vi "ConfigAndGrabEdited.vi"() -> ()   [LabVIEW 2025]
uses:
  <vilib>/userDefined/High Color/IMAQdx.ctl
  <vilib>/vision/driver/IMAQdx.llb/IMAQdx Buffer Number Mode.ctl
  <vilib>/vision/driver/NI_Vision_Acquisition_Software.lvlib
  <resource>/objmgr/imaqdx.rc
panel:
  in  "milliseconds to wait":u32
  in  "Packet size":i64=1 min=1 step=1
  out "DeviceModelName":string
  in  "OffsetY":i64=100
  in  "Height":i64=600 min=1 max=1088 step=1
  in  "OffsetX":i64=200
  in  "Width":i64=800 min=1 max=2048 step=1
  in  "ExposureTime (ms)":dbl=850.5 min=0.0 format="%#_9f"
  in  "Camera Name":T1
  out "Frame Rate":dbl(knob) scale=0.0..100.0 scale format="%.1f"
  out "Buffer Number":u32
  out "Image":T2(plugin-control)
  in  "stop":bool
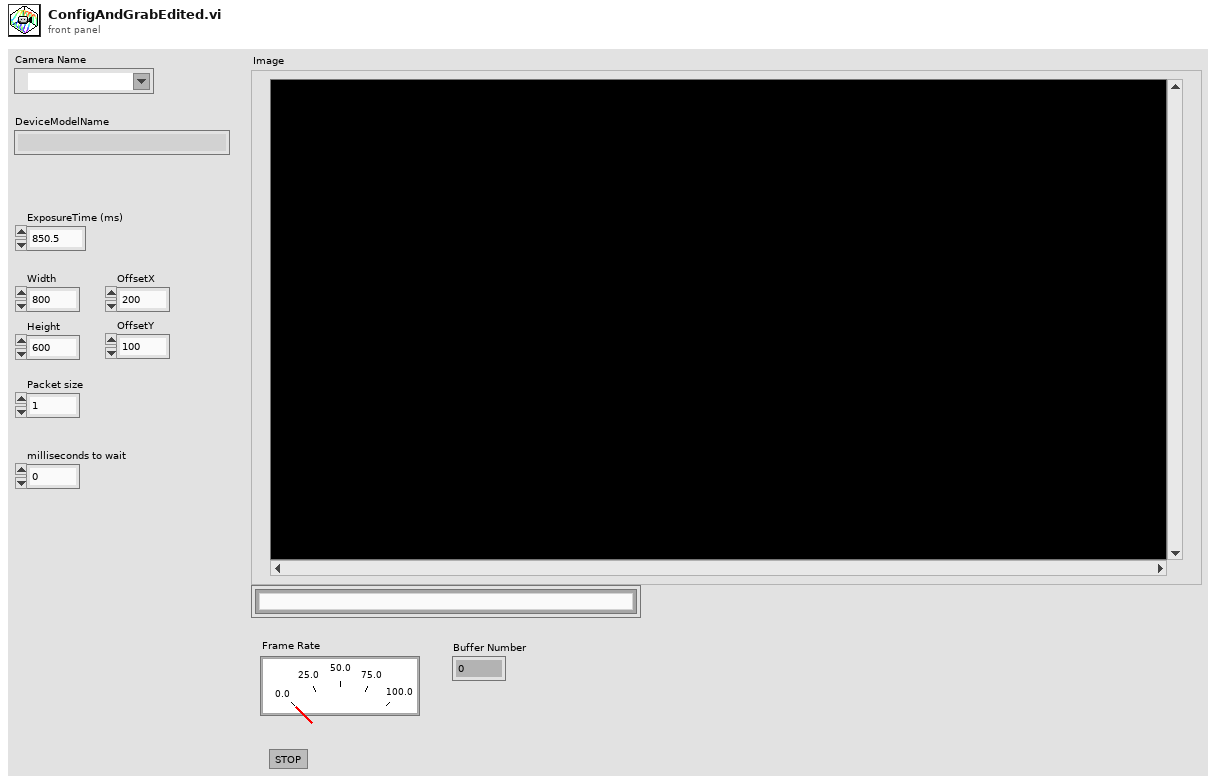
[diagram p1: front panel]
types:
  T1 = typedef "IMAQdx.ctl" = refnum<k21>
  T2 = typedef "IMAQ Image.ctl" = refnum<image>
  T3 = typedef "NI_Vision_Acquisition_Software.lvlib/IMAQdx Buffer Number Mode.ctl" = enum32{"Next", "Last", "Buffer Number", "Every", "Last New"}
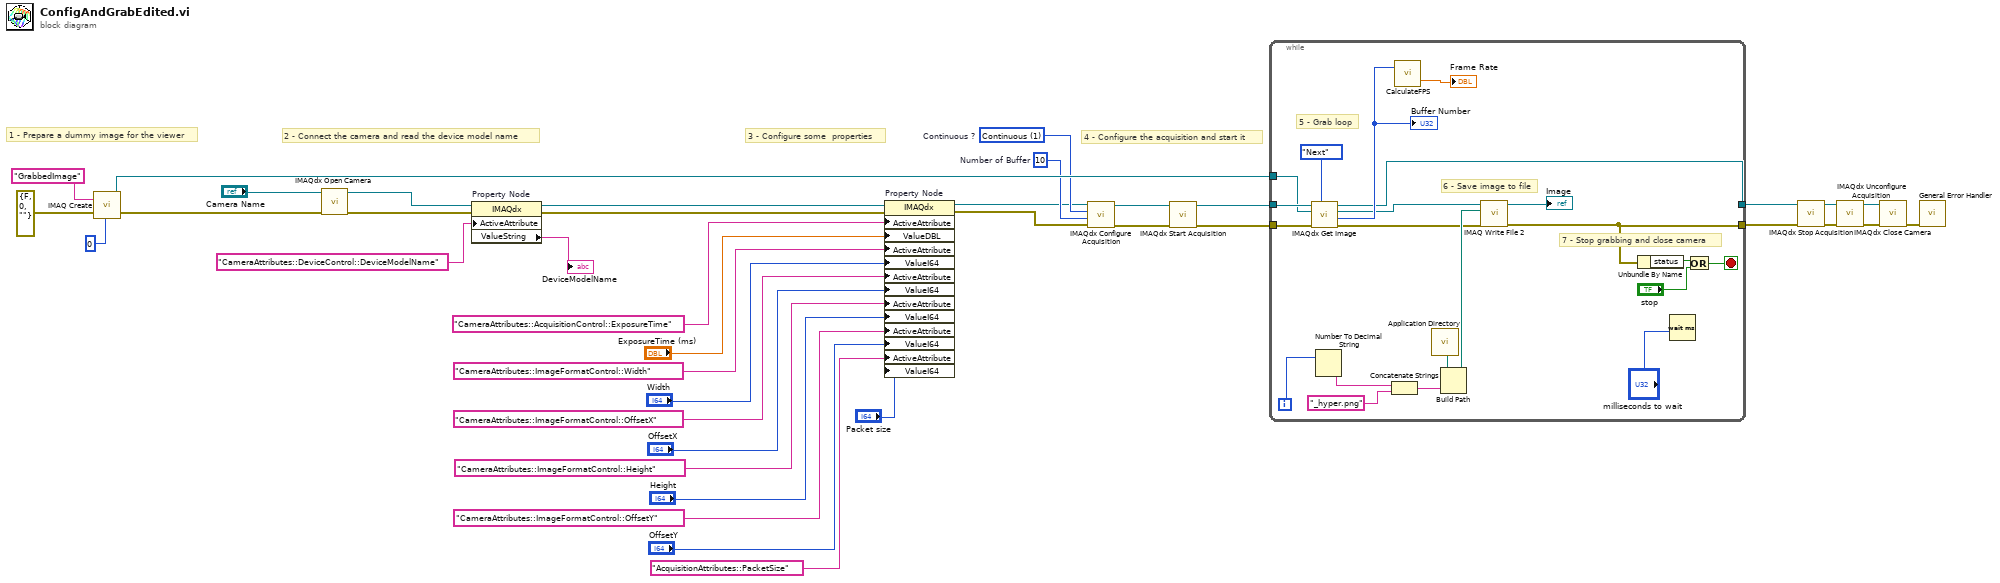
[diagram p0: block diagram]
diagram:
  w21 = u32 10  # Number of Buffer
  w20 = u32 1 items=["One Shot", "Continuous"]  # Continuous ?
  # "4 - Configure the acquisition and start it"
  # "3 - Configure some  properties"
  # "2 - Connect the camera and read the device model name"
  # "1 - Prepare a dummy image for the viewer"
  n1 = call "IMAQ Create"("Image Name"="GrabbedImage", "Image Type"=0, "error in (no error)"=errorcluster {"status"=FALSE, "code"=0, "source"=""}) -> ("New Image"=w24:T2, "error out"=w25:errorcluster)  [unwired: 1 in, 1 out]
  n2 = call <vilib>:"IMAQdx Open Camera.vi"("error in"=w25, "Session In"="Camera Name") -> ("error out"=w6:errorcluster, "Session Out"=w22:T1)  [unwired: 8 in]
  n3 = property on="Property Node" class="IMAQdx"(reference=w22, error in=w6, "ActiveAttribute"="CameraAttributes::DeviceControl::DeviceModelName") -> (reference out=w7:T1, error out=w5:errorcluster, "ValueString"=→"DeviceModelName":string)
  n4 = property on="Property Node" class="IMAQdx"(reference=w7, error in=w5, "ActiveAttribute"="CameraAttributes::AcquisitionControl::ExposureTime", "ValueDBL"="ExposureTime (ms)", "ActiveAttribute"="CameraAttributes::ImageFormatControl::Width", "ValueI64"="Width", "ActiveAttribute"="CameraAttributes::ImageFormatControl::OffsetX", "ValueI64"="OffsetX", "ActiveAttribute"="CameraAttributes::ImageFormatControl::Height", "ValueI64"="Height", "ActiveAttribute"="CameraAttributes::ImageFormatControl::OffsetY", "ValueI64"="OffsetY", "ActiveAttribute"="AcquisitionAttributes::PacketSize", "ValueI64"="Packet size") -> (reference out=w19:T1, error out=w18:errorcluster)
  n5 = call <vilib>:"IMAQdx Configure Acquisition.vi"("error in"=w18, "Number of Buffers"=w21, "Continuous?"=w20, "Session In"=w19) -> ("error out"=w39:errorcluster, "Session Out"=w38:T1)  [unwired: 6 out]
  n6 = call <vilib>:"IMAQdx Start Acquisition.vi"("error in"=w39, "Session In"=w38) -> ("error out"=w37:errorcluster, "Session Out"=w36:T1)  [unwired: 8 out]
  n7 = while {
    tunnel: w37 -> [w59]
    tunnel: w36 -> [w60]
    tunnel: w24 -> [w55]
    tunnel: [w41] -> w30
    tunnel: [w52] -> w29
    i -> [w48]
    stop <- w53 stop-if-true
    # "6 - Save image to file"
    # "7 - Stop grabbing and close camera"
    # "5 - Grab loop"
    n8 = call <vilib>:"IMAQdx Get Image.vi"("Buffer Number Mode (Next)"=IMAQdx_Buffer_Number_Mode."Next", "error in"=w59, "Image In"=w55, "Session In"=w60) -> ("error out"=w42:errorcluster, "Buffer Number Out"=w56:u32, "Image Out"=w50:T2, "Session Out"=w52:T1)  [unwired: 4 in]
    "Buffer Number" <- w56
    n9 = Number To Decimal String(number=w48) -> (decimal integer string=w45:string)  [unwired: 1 in]
    n10 = Concatenate Strings(w45, "_hyper.png") -> (w43:string)
    n11 = call "CalculateFPS.vi"("buffer number"=w56) -> ("processed FPS"=→"Frame Rate":dbl)  [unwired: 2 out]
    n12 = call <vilib>:"Application Directory.vi"() -> ("Application Directory"=w49:path)
    n13 = Build Path(base path=w49, name or relative path=w43) -> (appended path=w47:path)
    n14 = call-poly "IMAQ Write File 2"("error in (no error)"=w42, "File Path"=w47, "Image"=w50) -> ("error out"=w41:errorcluster, "Image Out (duplicate)"=→"Image":T2)  [unwired: 7 in]
    n15 = Unbundle By Name(w41) -> ("status"=w54:bool)
    n16 = Wait (ms)(milliseconds to wait="milliseconds to wait") -> ()  [unwired: 1 out]
    n17 = Or(x=w54, y="stop") -> (x .or. y?=w53:bool)
  }
  n18 = call <vilib>:"IMAQdx Stop Acquisition.vi"("error in"=w30, "Session In"=w29) -> ("error out"=w34:errorcluster, "Session Out"=w33:T1)  [unwired: 8 out]
  n19 = call <vilib>:"IMAQdx Unconfigure Acquisition.vi"("error in"=w34, "Session In"=w33) -> ("error out"=w31:errorcluster, "Session Out"=w32:T1)  [unwired: 8 out]
  n20 = call <vilib>:"IMAQdx Close Camera.vi"("error in"=w31, "Session In"=w32) -> ("error out"=w35:errorcluster)  [unwired: 9 out]
  n21 = call <vilib>:"General Error Handler.vi"("error in (no error)"=w35) -> ()  [unwired: 2 in, 13 out]
